vi "Append Relative Path String.vi"(10 "Relative Path":string, 11 "Base Path":path) -> (3 "Absolute Path":path)   [LabVIEW 2011, in "LVH-Toolbox.lvlib" / "LVH-Common.lvlib"]
doc: "Build an absolute path from a bath path and a relative path string. \nThis VI strips slashes from relative path and there is platform agnostic."
uses:
  LVH-Common.lvlib
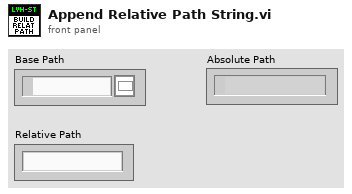
[diagram p1: front panel]
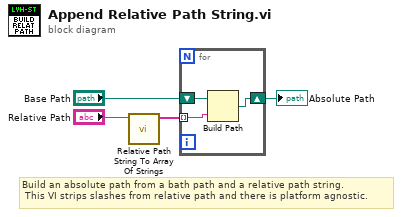
[diagram p0: block diagram]
diagram:
  # "Build an absolute path from a bath path and a relative path string. \n This VI strips slashes from relative path and there is platform agnostic."
  n1 = call "Relative Path String To Array Of Strings.vi"("Relative Path"="Relative Path") -> ("Relative Path Array"=w2:string[])  [unwired: 10 in]
  n2 = for {
    shift-right: [w5] -> w1
    shift-left: "Base Path" -> [w7]
    tunnel: w2 -> [w6] mode=indexing
    n3 = Build Path(base path=w7, name or relative path=w6) -> (appended path=w5:path)
  }
  "Absolute Path" <- w1
